vi "SendLocalMsg.vi"(0 "reference in":refnum<class "MessageAMC.lvclass">, 1 "receiver process":string, 5 "name":string, 7 "value":string, 9 "timeout (25000 ms)":i32=25000, 11 "error in (no error)":errorcluster) -> (4 "reference out":refnum<class "MessageAMC.lvclass">, 10 "timed out?":bool, 15 "error out":errorcluster)   [LabVIEW 2019, in "MessageAMC.lvclass"]
uses:
  MessageAMC.lvclass
  MessageAMC.lvclass/MessageAMC.ctl
  <vilib>/NI/AMC/Create Single Message.vi
  <vilib>/NI/AMC/Update Message Routing Info.vi
  <vilib>/NI/AMC/Send Message.vi
  <vilib>/NI/AMC/AMC.lvlib
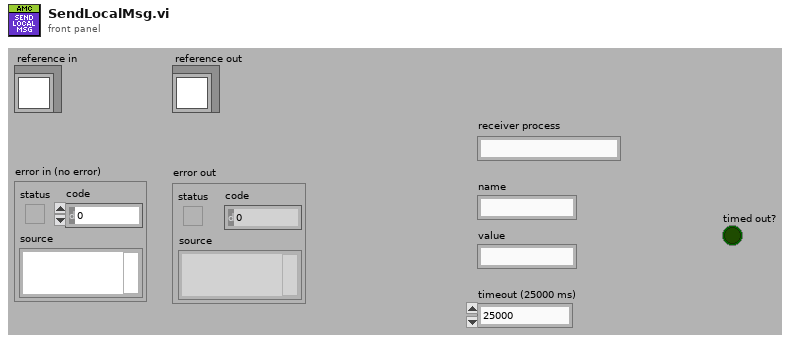
[diagram p1: front panel]
types:
  T1 = typedef "AMC.lvlib/Message Queue.ctl" = refnum<queue>
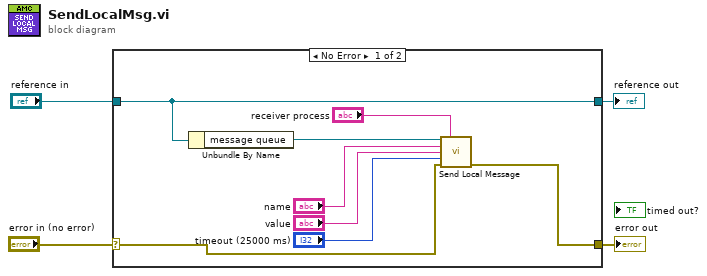
[diagram p0: block diagram]
diagram:
  n1 = case shown="No Error" "error in (no error)" {
    selector: "error in (no error)" -> [w12 w14]
    tunnel: [w10 w14] -> w3
    tunnel: [w5 w13] -> w1
    tunnel: "reference in" -> [w5 w13]
    frame No Error {
      n2 = Unbundle By Name(w5) -> ("message queue"=w11:T1)
      n3 = call <vilib>:"Send Local Message.vi"("message queue in"=w11, "receiver process (\"\" - local)"="receiver process", "message name"="name", "message value"="value", "timeout (-1 ms)"="timeout (25000 ms)", "error in"=w12) -> ("error out"=w10:errorcluster)  [unwired: 7 in, 2 out]
    }
    frame Error {
    }
  }
  "error out" <- w3
  "reference out" <- w1
